vi "Lift and Clamp Motors Test.vi"() -> ()   [LabVIEW 2014]
panel:
  in  "Direction":enum16{"Stop", "Up", "Down"}(ring)
  out "Lift Encoder":T1
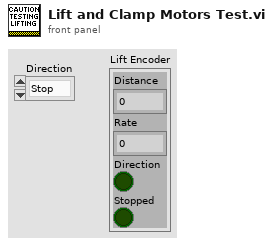
[diagram p1: front panel]
types:
  T1 = cluster{"Distance":dbl, "Rate":dbl, "Direction":bool, "Stopped":bool}
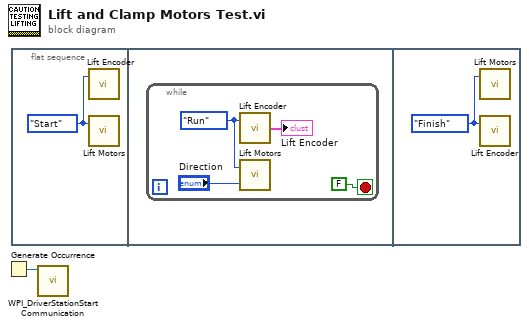
[diagram p0: block diagram]
diagram:
  n1 = Generate Occurrence() -> (w1:refnum<k4>)
  n2 = flat-sequence {
    frame #0 {
      w2 = enum8{"Start", "Run", "Finish"}."Start" ("Mode")
      n3 = call "Lift Encoder.vi"("Mode"=w2) -> ()  [unwired: 1 in, 1 out]
      n4 = call "Lift Motors.vi"("Mode"=w2) -> ()  [unwired: 2 in]
    }
    frame #1 {
      n5 = while {
        stop <- FALSE stop-if-true
        w5 = enum8{"Start", "Run", "Finish"}."Run" ("Mode")
        n6 = call "Lift Encoder.vi"("Mode"=w5) -> ("Lift Encoder"=→"Lift Encoder":T1)  [unwired: 1 in]
        n7 = call "Lift Motors.vi"("Direction"="Direction", "Mode"=w5) -> ()  [unwired: 1 in]
      }
    }
    frame #2 {
      w7 = enum8{"Start", "Run", "Finish"}."Finish" ("Mode")
      n8 = call "Lift Motors.vi"("Mode"=w7) -> ()  [unwired: 2 in]
      n9 = call "Lift Encoder.vi"("Mode"=w7) -> ()  [unwired: 1 in, 1 out]
    }
  }
  n10 = call <vilib>:"WPI_DriverStationStart Communication.vi"("occurrence"=w1) -> ()  [unwired: 11 in]
